vi "Flatten.vi"(8 "error in (no error)":errorcluster, 10 "Pretty Print?":bool, 11 "JSON Running Mean in":refnum<class "JSON Running Mean.lvclass">) -> (0 "error out":errorcluster, 2 "<JSON>":string)   [LabVIEW 2020, in "Library Commun.lvlib" / "JSON Running Mean.lvclass"]
uses:
  JSON Running Mean.lvclass
  JSON Value/JSON Value.lvclass
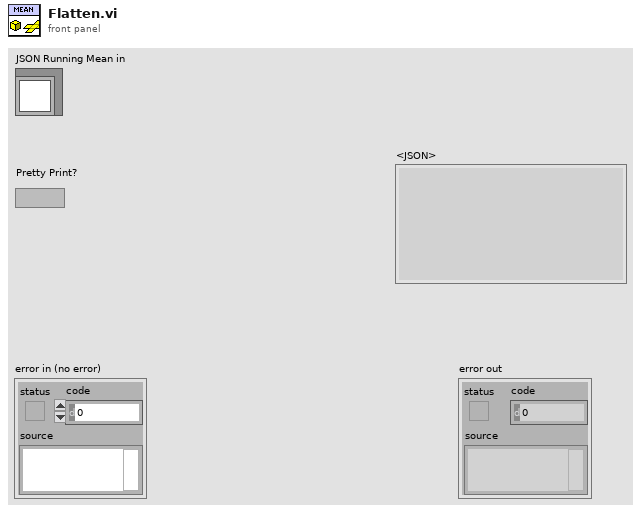
[diagram p1: front panel]
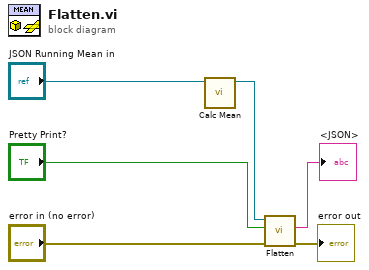
[diagram p0: block diagram]
diagram:
  n1 = call-dynamic "Calc Mean.vi"("JSON Statistics in"="JSON Running Mean in") -> ("JSON Value"=w5:refnum<class "JSON Value.lvclass">)  [unwired: 10 in]
  n2 = call-dynamic "Flatten.vi"("error in (no error)"="error in (no error)", "Pretty Print?"="Pretty Print?", "JSON Value in"=w5) -> ("error out"=→"error out":errorcluster, "<JSON>"=→"<JSON>":string)  [unwired: 7 in]
